vi "Basic RESTws.vi"() -> ()   [LabVIEW 2023]
uses:
  controls/MLA Loops.ctl
  controls/WebSocket VIG States.ctl
  Log/Log_Level.ctl
  API Message/API Message.lvclass
  WebSocket/WebSocket.lvclass
  <vilib>/Utility/config.llb/Write Key (Boolean).vi
  Request/Get Request.vi
  <vilib>/Utility/config.llb/Read Key (Double).vi
  <vilib>/Utility/config.llb/Write Key (String).vi
  <vilib>/addons/control/pid/pid.llb/PID (DBL).vi
  <vilib>/httpClient/POSTBuffer.vi
  Request/Request.lvclass
  Response/Response.lvclass
  MLA/MLA.lvclass
  <vilib>/Utility/config.llb/NI_LVConfig.lvlib
  Log/Log.lvclass
  Server/Server.lvclass
  <vilib>/httpClient/LabVIEWHTTPClient.lvlib
  <vilib>/addons/control/pid/NI_PID_pid.lvlib
panel:
  in  "Get Temperature":bool
  out "Current Temperature":dbl
  in  "Get Target":bool
  out "Current Target":dbl
  in  "Target Set":dbl
  in  "Get Ambient":bool
  in  "Get PIDs":bool
  out "Current Ambient":dbl
  out "Current PIDs":cluster{"P":dbl, "I":dbl, "D":dbl}
  in  "Ambient Set":dbl
  in  "PID Set":cluster{"P":dbl, "I":dbl, "D":dbl}={"P"=1.0, "I"=0.01, "D"=0.0}
  out "Target":dbl=23.0
  out "Ambient":dbl=23.0
  out "PID gains":cluster{"P":dbl, "I":dbl, "D":dbl}={"P"=1.0, "I"=0.01, "D"=0.0}
  out "Temperature Chart":dbl(graph)=23.0
  out "Temperature":dbl=23.0 format="%.2f"
  out "P_heater":dbl format="%.2f"
  in  "REST Send":bool
  in  "REST TX":string
  in  "WS Send":bool
  in  "WS TX":string
  out "All Messages":string
  out "Version":string="1.0.0" caption="V"
  out "Happy":bool=TRUE
  in  "ErrorButton":bool=TRUE
  out "Errors":bool
  out "Status":string="Initializing... "
  # "REST.ws Basic Example"
  # "REST Endpoints"
  # "Process Simulation"
  # "Write Enpoints - change Plant Values"
  # "Read Enpoints - retrieve Plant Values"
  # "All Messages"
  # "www.s5solutions.com"
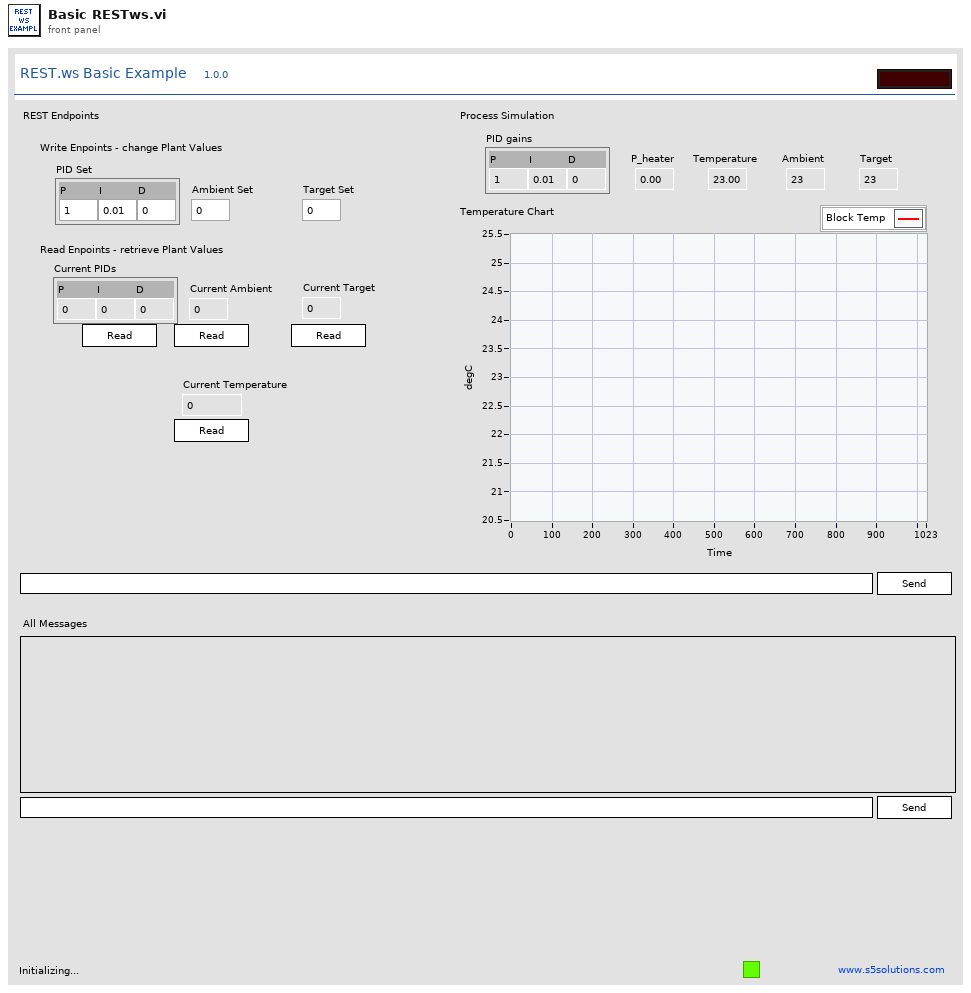
[diagram p1: front panel]
types:
  T1 = cluster{"proportional gain (Kc)":dbl, "integral time (Ti, min)":dbl, "derivative time (Td, min)":dbl}
  T2 = typedef "Log.lvclass/Log_Level.ctl" = enum16{"none", "info", "trace", "warn", "error", "fatal"}
  T3 = typedef "MLA Loops.ctl" = enum16{"Process", "REST", "WS"}
  T4 = typedef "WebSocket VIG States.ctl" = enum16{"Open", "Close", "Send", "Receive", "Check"}
  T5 = enum32{"invalid app kind", "Development System", "Run Time System", "Student Edition", "Embedded LabVIEW", "Evaluation", "Custom"}
  T6 = typedef "NI_LVConfig.lvlib/Config Data RefNum.ctl" = refnum<k1>
  T7 = typedef "LabVIEWHTTPClient.lvlib/ClientHandle.ctl" = refnum<k1>
  T8 = typedef "Request.ctl" = cluster{"Method":string, "URI":string, "Protocol":string, "Raw Path":string, "Query":string, "Fragment":string, "Raw Body":string, "Headers":variant, "Parameters":variant, "Body":variant, "Raw Header":string, "Path":string[]}
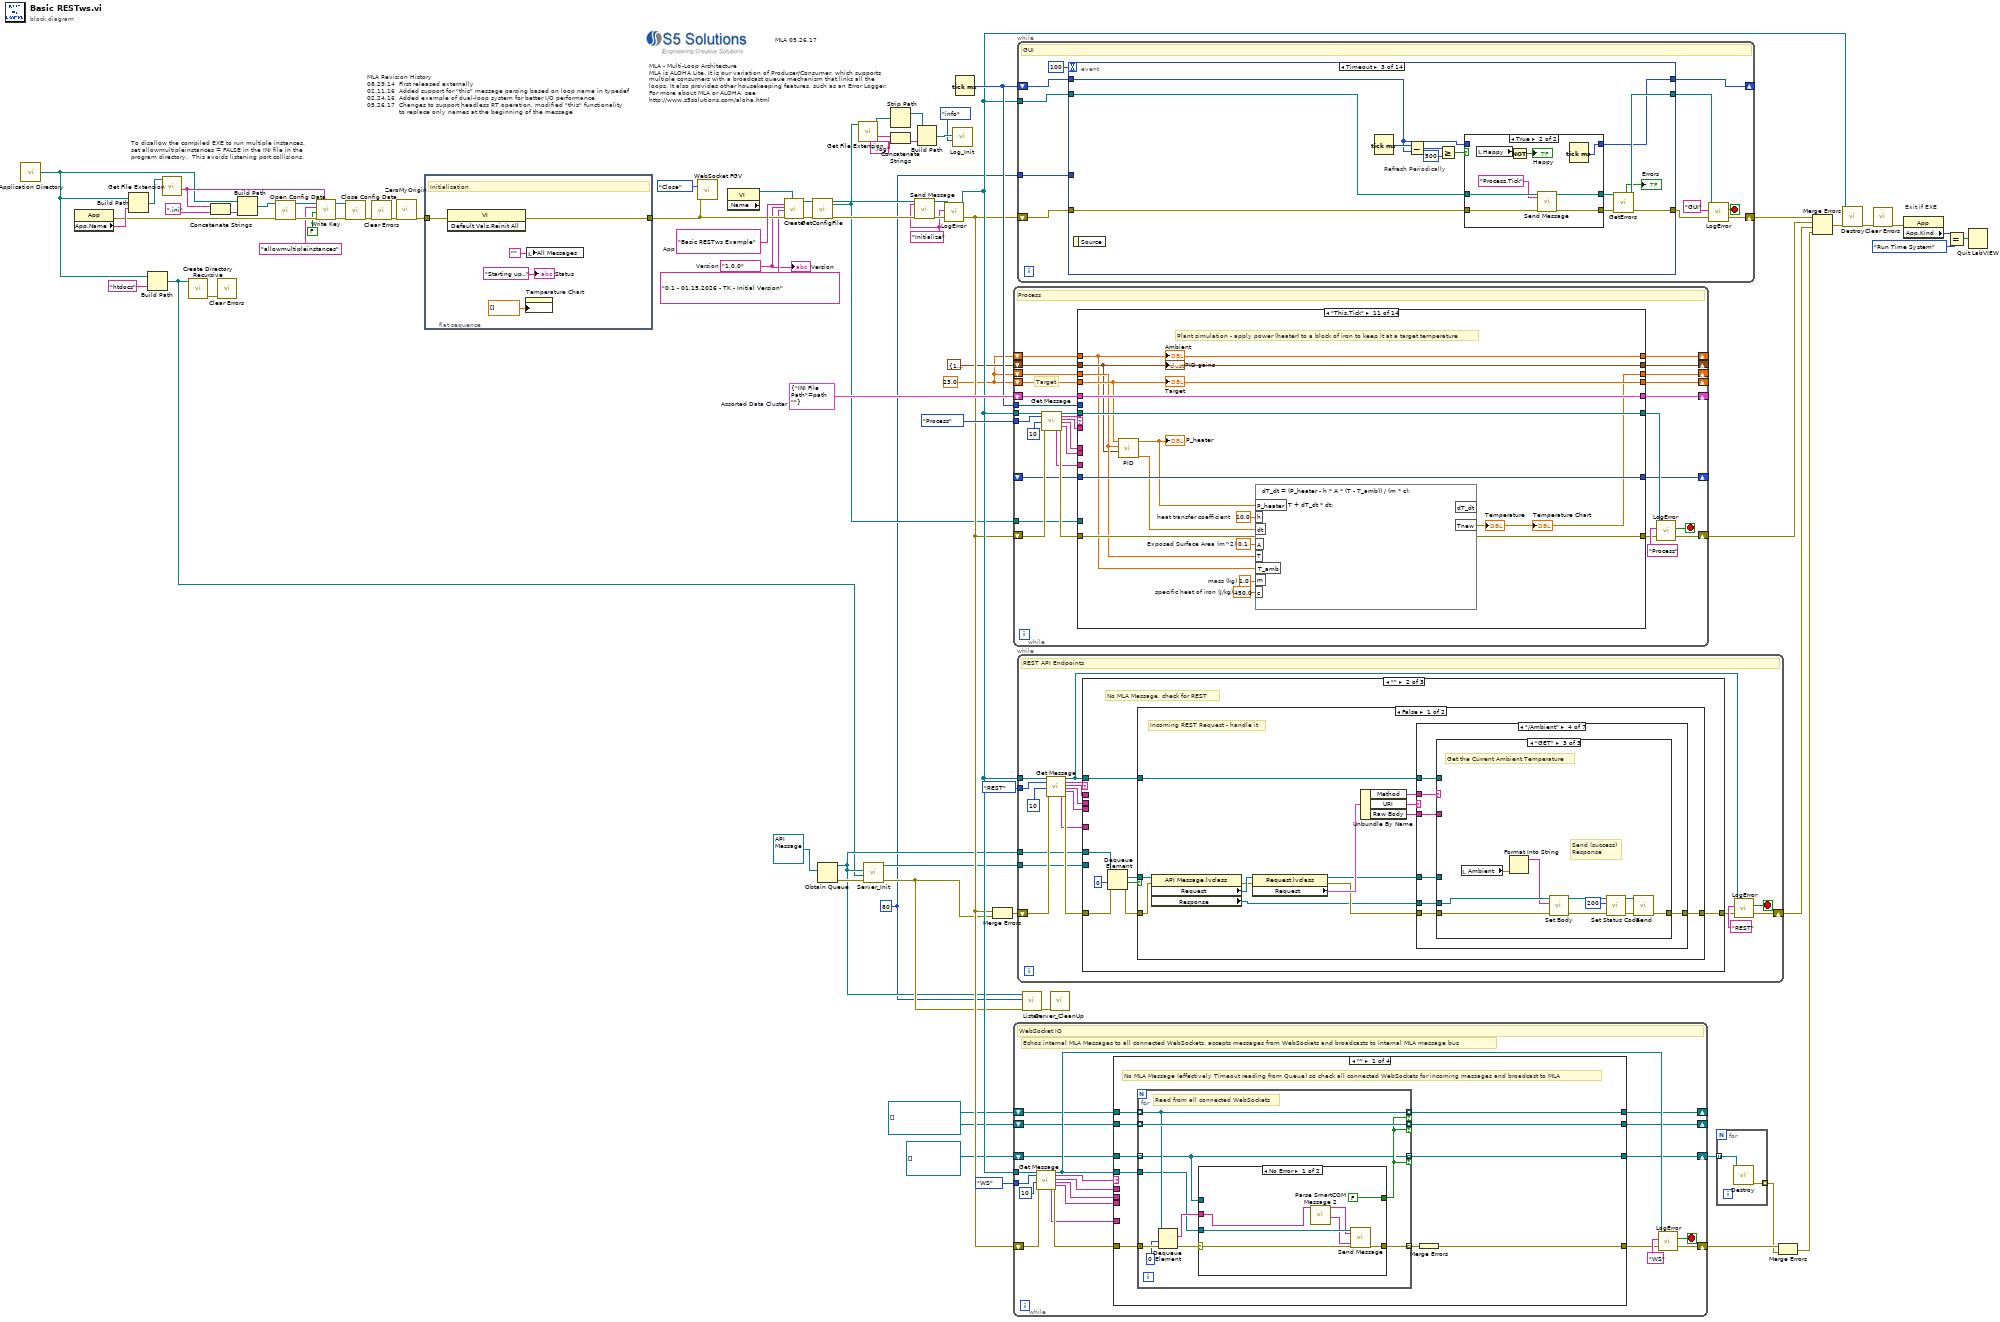
[diagram p0: block diagram]
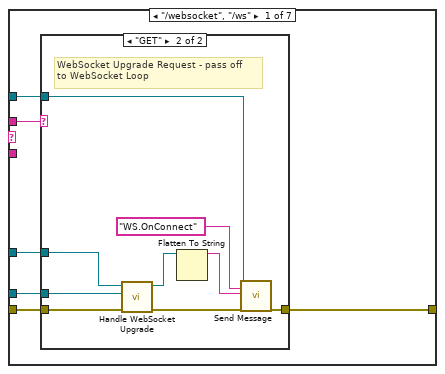
[diagram p3: hidden frame]
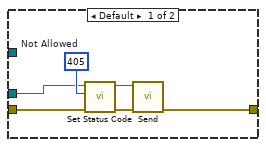
[diagram p4: hidden frame]
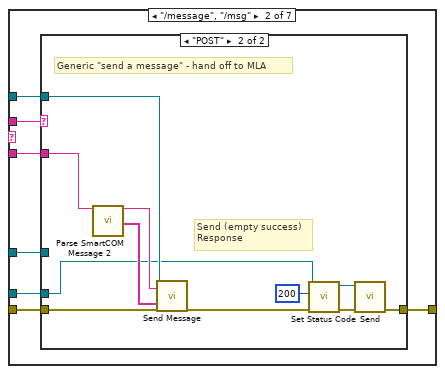
[diagram p5: hidden frame]
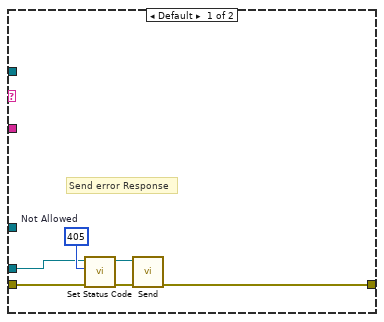
[diagram p6: hidden frame]
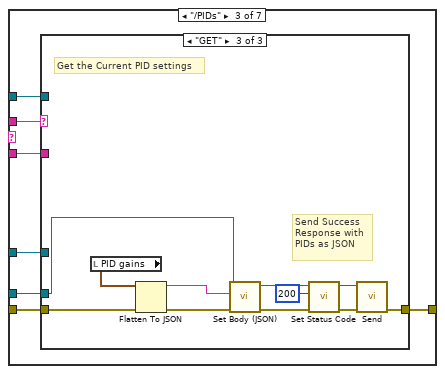
[diagram p7: hidden frame]
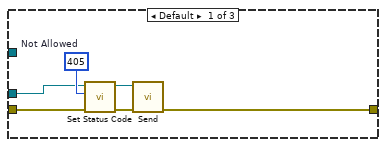
[diagram p8: hidden frame]
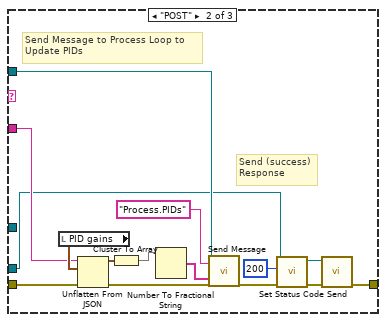
[diagram p9: hidden frame]
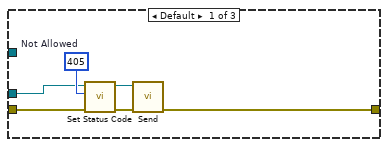
[diagram p10: hidden frame]
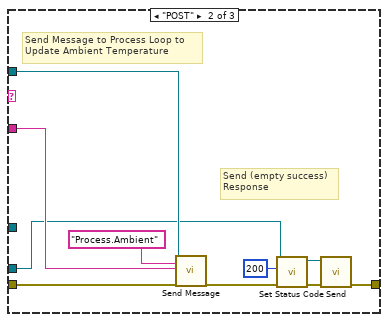
[diagram p11: hidden frame]
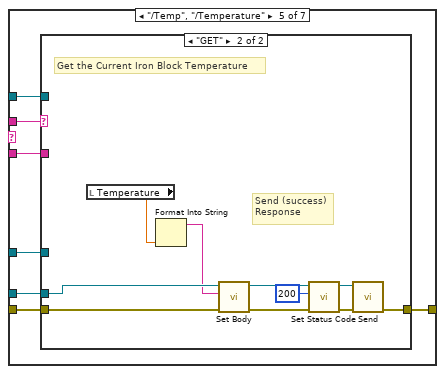
[diagram p12: hidden frame]
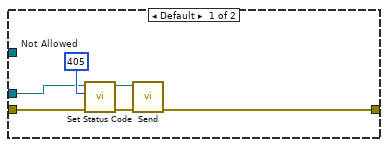
[diagram p13: hidden frame]
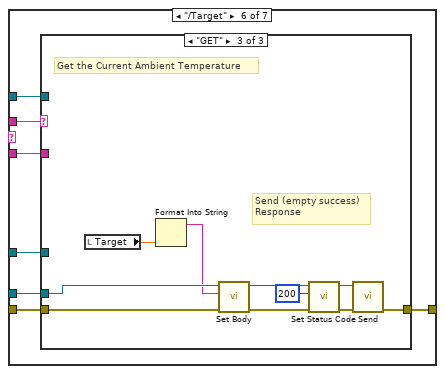
[diagram p14: hidden frame]
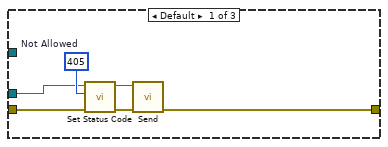
[diagram p15: hidden frame]
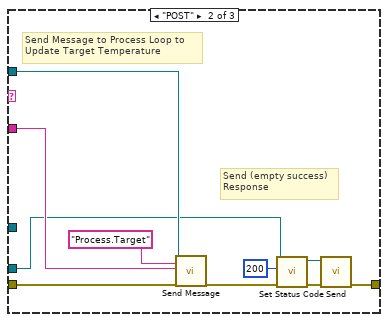
[diagram p16: hidden frame]
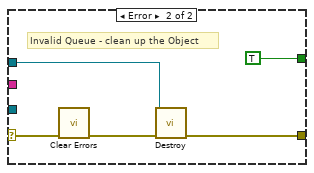
[diagram p20: hidden frame]
diagram:
  w7 = u16 80 ("Listen Port (80)")
  w12 = refnum<queue>[] []
  w5 = 23.0 ("Param 1")
  w42 = "1.0.0"  # Version
  w61 = cluster{"INI File Path":path} {"INI File Path"=path ""}  # Assorted Data Cluster
  w68 = "Basic RESTws Example"  # App
  w9 = "Initialize" ("element")
  # "To disallow the compiled EXE to run multiple instances,\nset allowmultipleinstances = FALSE in the INI file in the\nprogram directory.  This avoids listening port collisions."
  # "MLA Revision History\n08.29.14  First released externally\n02.11.16  Added support for \"this\" message parsing based on loop name in typedef\n02.24.16  Added example of dual-loop system for better I/O performance\n05.26.17  Changes to support headless RT operation, modified \"this\" functionality \n                to replace only names at the beginning of the message"
  # "MLA 05.26.17"
  # "MLA - Multi-Loop Architecture\nMLA is ALOHA Lite. It is our variation of Producer/Consumer, which supports multiple consumers with a broadcast queue mechanism that links all the loops. It also provides other housekeeping features, such as an Error Logger.\nFor more about MLA or ALOHA, see \nhttp://www.s5solutions.com/aloha.html"
  # "Exit if EXE"
  n1 = call <vilib>:"Application Directory.vi"() -> ("Application Directory"=w25:path)
  n2 = property class="App"() -> (error out=w48:errorcluster, "App.Name"=w50:string)  [unwired: 2 in, 1 out]
  n3 = Build Path(base path=w25, name or relative path=w50) -> (appended path=w49:path)
  n4 = Build Path(base path=w25, name or relative path="htdocs" ("section")) -> (appended path=w4:path)
  n5 = call <vilib>:"Get File Extension.vi"("file"=w49) -> ("filename without extension"=w36:string)  [unwired: 6 in, 4 out]
  n6 = call <vilib>:"Create Directory Recursive.vi"("directory"=w4) -> ("error out"=w3:errorcluster)  [unwired: 4 in, 2 out]
  n7 = Concatenate Strings(w36, ".ini" ("section")) -> (w47:string)
  n8 = call <vilib>:"Clear Errors.vi"("error in (no error)"=w3) -> ()  [unwired: 5 in, 2 out]
  n9 = Build Path(base path=w25, name or relative path=w47) -> (appended path=w46:path)
  n10 = call <vilib>:"Open Config Data.vi"("error in (no error)"=w48, "configuration file path"=w46) -> ("error out"=w55:errorcluster, "refnum"=w56:T6)  [unwired: 7 in, 1 out]
  n11 = call-poly <vilib>:"Write Key.vi"("section"=w36, "error in (no error)"=w55, "value"=FALSE, "key"="allowmultipleinstances", "refnum"=w56) -> ("error out"=w58:errorcluster, "refnum out"=w57:T6)  [unwired: 4 in, 1 out]
  n12 = call <vilib>:"Close Config Data.vi"("error in (no error)"=w58, "refnum"=w57) -> ("error out"=w52:errorcluster)  [unwired: 8 in, 1 out]
  n13 = call <vilib>:"Clear Errors.vi"("error in (no error)"=w52) -> ("error out"=w32:errorcluster)  [unwired: 5 in, 1 out]
  n14 = call "ZeroMyOrigin.vi"("error in (no error)"=w32) -> ("error out"=w69:errorcluster)  [unwired: 18 in]
  n15 = flat-sequence "Initialization" {
    tunnel: w69 -> [w74]
    tunnel: [w75] -> w45
    frame #0 {
      # "Initialization"
      n16 = invoke class="VI" method="Default Vals.Reinit All"(error in=w74) -> (error out=w75:errorcluster)  [unwired: 2 in, 2 out]
      n17 = property on="Temperature Chart" class="WFChart (strict)"("History Data"=dbl[] []) -> ()  [unwired: 2 in, 2 out]
      n18 = local write "All Messages"("") -> ()
      "Status" <- "Starting up.." ("Status")
    }
  }
  n19 = call "WebSocket FGV.vi"("Action"=WebSocket_VIG_States."Close", "error in (no error)"=w45) -> ()  [unwired: 8 in, 6 out]
  n20 = property class="VI" props=["Name"]() -> (reference out=w65:refnum<vi>)  [unwired: 2 in, 2 out]
  n21 = call "Create.vi"("Application Name"=w68, "Application Version"=w42, "Revision History"="0.1 - 01.15.2026 - TK - Initial Version" ("Version"), "error in (no error)"=w45, "VI Reference"=w65) -> ("MLA"=w62:refnum<class "MLA.lvclass">, "error out"=w64:errorcluster)  [unwired: 13 in]
  n22 = call-dynamic "GetConfigFile.vi"("MLA"=w62, "error in (no error)"=w64) -> ("MLA"=w63:refnum<class "MLA.lvclass">, "Config File"=w8:path, "error out"=w59:errorcluster)  [unwired: 15 in]
  n23 = Obtain Queue(element data type=refnum<class "API Message.lvclass"> refnum ("API Message.lvclass")) -> (queue out=w20:refnum<queue>, error out=w27:errorcluster)  [unwired: 4 in, 1 out]
  n24 = call <vilib>:"Get File Extension.vi"("file"=w8) -> ("filename without extension"=w31:string, "dup file"=w30:path)  [unwired: 6 in, 3 out]
  n25 = call "Server_Init.vi"("error in (no error)"=w27, "Static Data Folder"=w4, "API Queue"=w20) -> ("error out"=w21:errorcluster, "reference out"=w19:refnum<class "Server.lvclass">)  [unwired: 7 in]
  n26 = Strip Path(path=w30) -> (stripped path=w29:path)  [unwired: 1 out]
  n27 = Concatenate Strings(w31, ".log" ("section")) -> (w35:string)
  n28 = call-dynamic "Send Message.vi"("MLA"=w63, "Message"=w9, "error in (no error)"=w59) -> ("MLA"=w10:refnum<class "MLA.lvclass">, "error out"=w11:errorcluster)  [unwired: 15 in]
  n29 = Build Path(base path=w29, name or relative path=w35) -> (appended path=w34:path)
  n30 = call "LogError.vi"("Error To Log"=w11, "Context (\"Error\")"=w9, "reference in"=w10) -> ("Cleaned Error"=w23:errorcluster, "reference out"=w40:refnum<class "MLA.lvclass">)  [unwired: 2 in, 1 out]
  n31 = call "Log_Init.vi"("Level"=Log_Level."info", "Log File"=w34) -> ()  [unwired: 8 in, 2 out]
  n32 = Tick Count (ms)() -> (millisecond timer value=w60:u32)
  n33 = Merge Errors(w23, w21) -> (w22:errorcluster)
  n34 = while "Process" {
    shift-right: [w103] -> w2
    shift-left: w23 -> [w100]
    tunnel: w40 -> [w101]
    tunnel: MLA_Loops."Process" ("Customize This Typedef =>") -> [w98]
    tunnel: w8 -> [w94]
    shift-right: [w92] -> _
    shift-left: w61 -> [w93]
    tunnel: w60 -> [w91]
    shift-right: [w89] -> _
    shift-left: _ -> [w90]
    shift-right: [w87] -> _
    shift-left: w5 -> [w86]
    shift-right: [w81] -> _
    shift-left: T1 {"proportional gain (Kc)"=1.0, "integral time (Ti, min)"=0.01, "derivative time (Td, min)"=0.0} ("PID gains") -> [w84]
    shift-right: [w82] -> _
    shift-left: w5 -> [w83]
    shift-right: [w80] -> _
    shift-left: w5 -> [w79]
    stop <- w96 stop-if-true
    # "Target"
    # "Process"
    n35 = call-dynamic "Get Message.vi"("MLA"=w101, "Loop"=w98, "Timeout (100mS)"=10, "error in (no error)"=w100) -> ("Raw Message"=w85:string, "MLA"=w97:refnum<class "MLA.lvclass">, "Message"=w104:string, "Param 1"=w108:string, "Param 2"=w107:string, "Params"=w106:string[], "error out"=w99:errorcluster)  [unwired: 8 in, 1 out]
    n36 = case shown="\"This.Tick\"" w104 {
      tunnel: [w116 w124 w134 w146 w155 w156 w170 w188 w208 w216 w231 w240 w249 w261] -> w102
      tunnel: w99 -> [w116 w124 w134 w141 w155 w156 w181 w196 w208 w216 w231 w240 w249 w261]
      tunnel: w108 -> [_ _ _ _ _ _ _ w190 _ _ _ w233 w243 _]
      tunnel: w107 -> [_ _ _ _ _ _ _ _ _ _ _ _ _ _]
      tunnel: w106 -> [_ _ _ _ _ _ _ _ _ _ _ _ _ w254]
      tunnel: w97 -> [w115 w123 w133 w145 w154 w157 w169 w194 w207 w215 w230 w239 w248 w260]
      tunnel: [w115 w123 w133 w144 w154 w157 w169 w187 w207 w215 w230 w239 w248 w260] -> w95
      tunnel: w94 -> [_ _ _ _ _ _ w173 _ _ _ _ _ _ _]
      tunnel: w93 -> [w114 w122 w136 w147 w153 w163 w174 w198 w206 w214 w229 w238 w247 w259]
      tunnel: [w114 w122 w136 w147 w153 w163 w165 w198 w206 w214 w229 w238 w247 w259] -> w92
      tunnel: w91 -> [_ _ _ _ _ _ _ _ _ _ _ _ _ _]
      tunnel: w90 -> [w113 w121 w129 w143 w152 _ w172 w193 w205 w213 w228 w237 w246 w258]
      tunnel: [w113 w121 w129 w143 w152 0 w172 w193 w205 w213 w228 w237 w246 w258] -> w89
      tunnel: [w112 w120 w135 w142 w151 w161 w171 w189 w204 w212 w227 w236 w241 w257] -> w87
      tunnel: w86 -> [w112 w120 w135 w142 w151 w161 w171 w189 w204 w212 w227 w236 _ w257]
      tunnel: w85 -> [_ _ w130 _ _ _ _ _ _ _ _ _ _ _]
      tunnel: w84 -> [w111 w118 w128 w139 w150 w160 w168 w184 w203 w211 w223 w234 w244 w253]
      tunnel: w83 -> [w110 w119 w127 w138 w149 w159 w167 w183 w202 w210 w225 w235 w245 w256]
      tunnel: [w110 w119 w127 w138 w149 w159 w167 w183 w202 w210 w217 w235 w245 w256] -> w82
      tunnel: [w111 w118 w128 w139 w150 w160 w168 w184 w203 w211 w223 w234 w244 w250] -> w81
      tunnel: [w109 w117 w126 w137 w148 w158 w166 w182 w201 w209 w218 w232 w242 w255] -> w80
      tunnel: w79 -> [w109 w117 w126 w137 w148 w158 w166 w182 w201 w209 w218 _ w242 w255]
      frame "-----Miscellaneous-----" {
      }
      frame "" {
        # "No Message - do nothing"
      }
      frame Default {
        # "Unknown/Unhandled message, save it to the message log"
        n37 = local read "All Messages"() -> (w132:string)
        n38 = Concatenate Strings(w132, w130, "\r\n") -> (→"All Messages":string)
      }
      frame "Shutdown" {
        n39 = call "Shutdown.vi"("error in (no error)"=w141) -> ("error out"=w140:errorcluster)  [unwired: 10 in]
        n40 = call-dynamic "Stop.vi"("reference in"=w145, "error in (no error)"=w140) -> ("reference out"=w144:refnum<class "MLA.lvclass">, "error out"=w146:errorcluster)  [unwired: 16 in]
      }
      frame "-----Setup-----" {
      }
      frame "Initialize" {
        n41 = local write "Status"("Initializing... " ("Status")) -> ()
      }
      frame "This.LoadCurrentINI" {
        n42 = call <vilib>:"Open Config Data.vi"("error in (no error)"=w181, "configuration file path"=w173) -> ("error out"=w180:errorcluster, "refnum"=w178:T6)  [unwired: 7 in, 1 out]
        n43 = call-poly <vilib>:"Read Key.vi"("section"="Sim", "error in (no error)"=w180, "key"="Target", "refnum"=w178) -> ("error out"=w177:errorcluster, "refnum out"=w175:T6)  [unwired: 4 in, 2 out]
        n44 = call <vilib>:"Close Config Data.vi"("error in (no error)"=w177, "refnum"=w175) -> ("error out"=w170:errorcluster)  [unwired: 8 in, 1 out]
        n45 = Bundle By Name(cluster=w174, "INI File Path"=w173) -> (w165:cluster{"INI File Path":path})
      }
      frame "This.UpdateINI" {
        n46 = call "Clear Component Lists.vi"("error in (no error)"=w196, "MLA in"=w194) -> ("error out"=w195:errorcluster, "MLA out"=w187:refnum<class "MLA.lvclass">)  [unwired: 8 in]
        n47 = Unbundle By Name(w198) -> ("INI File Path"=w197:path)
        n48 = call <vilib>:"Open Config Data.vi"("error in (no error)"=w195, "configuration file path"=w197) -> ("error out"=w191:errorcluster, "refnum"=w192:T6)  [unwired: 7 in, 1 out]
        n49 = call-poly <vilib>:"Write Key.vi"("section"="Sim", "error in (no error)"=w191, "value"=w190, "key"="Target", "refnum"=w192) -> ("error out"=w185:errorcluster, "refnum out"=w186:T6)  [unwired: 4 in, 1 out]
        n50 = call <vilib>:"Close Config Data.vi"("error in (no error)"=w185, "refnum"=w186) -> ("error out"=w188:errorcluster)  [unwired: 8 in, 1 out]
      }
      frame "-----Menu Functions-----" {
      }
      frame "-----Manage Data-----" {
      }
      frame "This.Tick" {
        w219 = 450.0  # specific heat of iron (J/kg)
        w220 = 1.0  # mass (kg)
        w221 = 0.1  # Exposed Surface Area (m^2)
        w222 = 10.0  # heat transfer coefficient
        # "Plant simulation - apply power (heater) to a block of iron to keep it at a target temperature"
        n51 = call-poly <vilib>:"PID.vi"("PID gains"=w223, "process variable"=w225, "setpoint"=w227) -> ("dt out (s)"=w224:dbl, "output"=w226:dbl)  [unwired: 7 in]
        "P_heater" <- w226
        n52 = formula code="dT_dt = (P_heater - h * A * (T - T_amb)) / (m * c);\n\nTnew = T + dT_dt * dt;"("P_heater"=w226, "h"=w222, "A"=w221, "T"=w225, "T_amb"=w218, "m"=w220, "c"=w219, "dt"=w224) -> ("Tnew"=w217:dbl)  [unwired: 1 out]
        "Temperature Chart" <- w217
        "Temperature" <- w217
        "PID gains" <- w223
        "Ambient" <- w218
        "Target" <- w227
      }
      frame "This.Ambient" {
        n53 = Scan From String(input string=w233) -> (output 1=w232:dbl)  [unwired: 4 in, 3 out]
      }
      frame "This.Target" {
        n54 = Scan From String(input string=w243) -> (output 1=w241:dbl)  [unwired: 4 in, 3 out]
      }
      frame "This.PIDs" {
        n55 = Cluster To Array(cluster=w253) -> (array=w252:dbl[])
        n56 = for {
          tunnel: w254 -> [w264] mode=indexing
          tunnel: w252 -> [w263] mode=indexing
          tunnel: [w262] -> w251 mode=indexing
          n57 = Fract/Exp String To Number(string=w264, default (0 dbl)=w263) -> (number=w262:dbl)  [unwired: 2 in, 1 out]
        }
        n58 = Array To Cluster(array=w251) -> (cluster=w250:cluster{"[0]":dbl, "[1]":dbl, "[2]":dbl})
      }
    }
    n59 = call "LogError.vi"("Error To Log"=w102, "Context (\"Error\")"="Process" ("Context"), "reference in"=w95) -> ("Cleaned Error"=w103:errorcluster, "Stop?"=w96:bool)  [unwired: 2 in, 1 out]
  }
  n60 = while "Send to RT" {
    shift-right: [w284] -> w16
    shift-left: w23 -> [w277]
    tunnel: MLA_Loops."WS" ("Loop") -> [w283]
    tunnel: w40 -> [w282]
    shift-right: [w271] -> w17
    shift-left: refnum<class "WebSocket.lvclass">[] [] -> [w272]
    shift-right: [w266] -> _
    shift-left: w12 -> [w268]
    shift-right: [w267] -> _
    shift-left: w12 -> [w269]
    stop <- w275 stop-if-true
    # "Echos internal MLA Messages to all connected WebSockets, accepts messages from WebSockets and broadcasts to internal MLA message bus"
    # "WebSocket IO"
    n61 = call-dynamic "Get Message.vi"("MLA"=w282, "Loop"=w283, "Timeout (100mS)"=10, "error in (no error)"=w277) -> ("Raw Message"=w274:string, "MLA"=w273:refnum<class "MLA.lvclass">, "Message"=w281:string, "Param 1"=w280:string, "Param 2"=w279:string, "Params"=w278:string[], "error out"=w276:errorcluster)  [unwired: 8 in, 1 out]
    n62 = case shown="\"\"" w281 {
      tunnel: w276 -> [w294 w322 w340 w346]
      tunnel: [w286 w318 w329 w343] -> w265
      tunnel: w280 -> [_ _ w342 w344]
      tunnel: w279 -> [_ _ _ _]
      tunnel: w278 -> [_ _ _ _]
      tunnel: w273 -> [w287 _ _ _]
      tunnel: w274 -> [_ w319 _ _]
      tunnel: w272 -> [w295 w324 w339 w349]
      tunnel: [w293 w324 w338 w350] -> w271
      tunnel: w269 -> [w291 w323 w335 w352]
      tunnel: w268 -> [w290 w321 w334 w351]
      tunnel: [w289 w323 w331 w347] -> w267
      tunnel: [w288 w321 w330 w348] -> w266
      frame "" {
        # "No MLA Message (effectively Timeout reading from Queue) so check all connected WebSockets for incoming messages and broadcast to MLA"
        n63 = for {
          tunnel: w295 -> [w298] mode=indexing
          tunnel: w294 -> [w304]
          tunnel: [w298] -> w293 mode=indexing if=w299
          tunnel: [w300] -> w292 mode=indexing
          tunnel: w291 -> [w303] mode=indexing
          tunnel: w290 -> [w305] mode=indexing
          tunnel: [w303] -> w289 mode=indexing if=w299
          tunnel: [w305] -> w288 mode=indexing if=w299
          tunnel: w287 -> [w296]
          # "Read from all connected WebSockets"
          n64 = Dequeue Element(queue=w303, timeout in ms (-1)=0, error in (no error)=w304) -> (element=w302:string, error out=w301:errorcluster)  [unwired: 2 out]
          n65 = case shown="No Error" w301 {
            selector: w301 -> [w311 w317]
            tunnel: w302 -> [w308 _]
            tunnel: [w310 w314] -> w300
            tunnel: [FALSE TRUE] -> w299
            tunnel: w298 -> [_ w313]
            tunnel: w296 -> [w309 _]
            frame No Error {
              n66 = call "Parse SmartCOM Message 2.vi"("Message"=w308) -> ("Root Message"=w307:string, "All Params"=w306:string[])  [unwired: 10 in, 7 out]
              n67 = call-dynamic "Send Message.vi"("MLA"=w309, "Message"=w307, "Params"=w306, "error in (no error)"=w311) -> ("error out"=w310:errorcluster)  [unwired: 14 in, 1 out]
            }
            frame Error {
              # "Invalid Queue - clean up the Object"
              n68 = call <vilib>:"Clear Errors.vi"("error in (no error)"=w317) -> ("error out"=w315:errorcluster)  [unwired: 5 in, 1 out]
              n69 = call-dynamic "Destroy.vi"("error in (no error)"=w315, "reference in"=w313) -> ("error out"=w314:errorcluster)  [unwired: 8 in, 1 out]
            }
          }
        }
        n70 = Merge Errors(w292) -> (w286:errorcluster)
      }
      frame Default {
        # "Unknown message - send to all connected WebSockets"
        n71 = for {
          tunnel: w322 -> [w327]
          tunnel: w321 -> [w326] mode=indexing
          tunnel: [w328] -> w320 mode=indexing
          tunnel: w319 -> [w325]
          n72 = Enqueue Element(queue=w326, element=w325, error in (no error)=w327) -> (error out=w328:errorcluster)  [unwired: 1 in, 2 out]
        }
        n73 = Merge Errors(w320) -> (w318:errorcluster)
      }
      frame "This.OnConnect" {
        # "Special Message indicating new connection from REST loop"
        n74 = Unflatten From String(type=refnum<class "WebSocket.lvclass"> refnum ("WebSocket"), binary string=w342, error in (no error)=w340) -> (value=w337:refnum<class "WebSocket.lvclass">, error out=w336:errorcluster)  [unwired: 2 in, 1 out]
        n75 = Build Array (concatenate)(w339, w337) -> (w338:refnum<class "WebSocket.lvclass">[])
        n76 = property class="WebSocket"(reference=w337, error in=w336) -> (error out=w329:errorcluster, "properties:FromSocket"=w333:refnum<queue>, "properties:ToSocket"=w332:refnum<queue>)  [unwired: 1 out]
        n77 = Build Array (concatenate)(w335, w333) -> (w331:refnum<queue>[])
        n78 = Build Array (concatenate)(w334, w332) -> (w330:refnum<queue>[])
      }
      frame "This.Transmit" {
        # "Special explicit message (not really needed because of the Default case) to send data to all connected WebSockets"
        n79 = for {
          tunnel: w352 -> [w358] mode=indexing
          tunnel: w351 -> [w354] mode=indexing
          tunnel: [w359] -> w350 mode=indexing
          tunnel: w349 -> [w359] mode=indexing
          tunnel: [w355] -> w348 mode=indexing
          tunnel: [w358] -> w347 mode=indexing
          tunnel: w346 -> [w356]
          tunnel: [w357] -> w345 mode=indexing
          tunnel: w344 -> [w353]
          n80 = Enqueue Element(queue=w354, element=w353, error in (no error)=w356) -> (queue out=w355:refnum<queue>, error out=w357:errorcluster)  [unwired: 1 in, 1 out]
        }
        n81 = Merge Errors(w345) -> (w343:errorcluster)
      }
    }
    n82 = call "LogError.vi"("Error To Log"=w265, "Context (\"Error\")"="WS" ("Context"), "reference in"=w273) -> ("Cleaned Error"=w284:errorcluster, "Stop?"=w275:bool)  [unwired: 2 in, 1 out]
  }
  n83 = while "GUI" {
    shift-right: [w368] -> w73
    shift-left: w23 -> [w370]
    shift-right: [w361] -> _
    shift-left: w60 -> [w366]
    tunnel: w40 -> [w363]
    tunnel: w7 -> [w360]
    stop <- w365 stop-if-true
    # "GUI"
    n84 = event shown="[2] Timeout" {
      selector: _ -> [_ _ _ _ _ _ _ _ _ _ _ _ _ _]
      dyn-events: _ -> [_ _ _ _ _ _ _ _ _ _ _ _ _ _]
      timeout: 100 -> [_ _ _ _ _ _ _ _ _ _ _ _ _ _]
      tunnel: w370 -> [w371 w382 w394 w426 w435 w441 w461 w476 w491 w506 w520 w534 w548 w559]
      tunnel: [w373 w380 w403 w426 w434 w442 w455 w471 w486 w501 w521 w535 w549 w558] -> w367
      tunnel: w366 -> [w376 w383 w395 w425 w436 w451 w467 w482 w497 w512 w527 w541 w555 w557]
      tunnel: [w376 w383 w397 w425 w436 w451 w467 w482 w497 w512 w527 w541 w555 w557] -> w361
      tunnel: w363 -> [w372 w381 w391 w424 w433 w448 w466 w481 w496 w511 w526 w540 w554 w556]
      tunnel: [w374 w379 w398 w424 w432 w448 w466 w481 w496 w511 w526 w540 w554 w556] -> w362
      tunnel: w360 -> [_ _ _ _ _ w439 w459 w474 w489 w504 w519 w533 w547 _]
      event Panel Close? {
        n85 = event-data() -> ()  [unwired: 1 in, 1 out]
        n86 = call-dynamic "Send Message.vi"("MLA"=w372, "Message"="Shutdown" ("element"), "error in (no error)"=w371) -> ("MLA"=w374:refnum<class "MLA.lvclass">, "error out"=w373:errorcluster)  [unwired: 15 in]
        n87 = event-data("Discard?"=TRUE) -> ()  [unwired: 1 in, 1 out]
      }
      event Menu Selection (User) {
        n88 = event-data() -> ("ItemTag"=w378:string)  [unwired: 1 in]
        n89 = disable-structure shown="Enabled" {
          disable-tunnel: w382 -> [w388 w389]
          disable-tunnel: w381 -> [w387 w390]
          disable-tunnel: [w386 w389] -> w380
          disable-tunnel: [w385 w390] -> w379
          disable-tunnel: w378 -> [w384 _]
          frame Enabled {
            n90 = call "Read Menu Action.vi"("error in (no error)"=w388, "ItemTag"=w384, "MLA in"=w387) -> ("error out"=w386:errorcluster, "MLA out"=w385:refnum<class "MLA.lvclass">)  [unwired: 7 in]
          }
          frame Disabled {
          }
        }
      }
      event Timeout {
        # "Refresh Periodically"
        n91 = event-data() -> ()  [unwired: 1 in, 1 out]
        n92 = Tick Count (ms)() -> (millisecond timer value=w400:u32)
        n93 = Subtract(x=w400, y=w395) -> (x-y=w401:u32)
        n94 = Greater Or Equal?(x=w401, y=u32 500) -> (x >= y?=w399:bool)
        n95 = case shown="True" w399 {
          tunnel: w395 -> [w406 _]
          tunnel: [w406 w412] -> w397
          tunnel: w394 -> [w404 w411]
          tunnel: [w404 w410] -> w393
          tunnel: w391 -> [w405 w409]
          tunnel: [w405 w408] -> w392
          frame False {
          }
          frame True {
            n96 = local read "Happy"() -> (w413:bool)
            n97 = Not(x=w413) -> (.not. x?=→"Happy":bool)
            n98 = call-dynamic "Send Message.vi"("MLA"=w409, "Message"="Process.Tick", "error in (no error)"=w411) -> ("MLA"=w408:refnum<class "MLA.lvclass">, "error out"=w410:errorcluster)  [unwired: 15 in]
            n99 = Tick Count (ms)() -> (millisecond timer value=w412:u32)
          }
        }
        n100 = call-dynamic "GetErrors.vi"("error in (no error)"=w393, "reference in"=w392) -> ("error out"=w403:errorcluster, "reference out"=w398:refnum<class "MLA.lvclass">, "Uncleared Errors"=→"Errors":bool)  [unwired: 4 in, 3 out]
      }
      event Key Down {
        n101 = event-data() -> ("Char"=w421:i16, "PlatMods.Ctrl"=w422:bool, "PlatMods.Shift"=w423:bool)  [unwired: 1 in]
        n102 = String To Byte Array(string="B") -> (unsigned byte array=w419:u8[])
        n103 = Index Array(array=w419) -> (element=w418:u8)  [unwired: 1 in]
        n104 = And(x=w422, y=w423) -> (x .and. y?=w416:bool)
        n105 = Equal?(x=w418, y=w421) -> (x = y?=w417:bool)
        n106 = And(x=w417, y=w416) -> (x .and. y?=w415:bool)
        n107 = case shown="True" w415 {
          frame False {
          }
          frame True {
            n108 = property class="VI"("BDWin.Open"=TRUE ("Block Diagram Window:Open")) -> ()  [unwired: 2 in, 2 out]
          }
        }
      }
      event "WS Send": Value Change {
        n109 = event-data() -> ()  [unwired: 1 in, 1 out]
        n110 = String Length(string="WS TX") -> (length=w428:i32)
        n111 = call-dynamic "Send Message.vi"("MLA"=w433, "Message"="WS.Transmit" ("element"), "Param 1"="WS TX", "error in (no error)"=w435) -> ("MLA"=w432:refnum<class "MLA.lvclass">, "error out"=w434:errorcluster)  [unwired: 14 in]
        n112 = property on="WS TX" class="Str"("Text.Selection End"=u32 0 ("Text.Selection:End"), "Text.Selection Start"=w428) -> ()  [unwired: 2 in, 2 out]
      }
      event "REST Send": Value Change {
        n113 = event-data() -> ()  [unwired: 1 in, 1 out]
        n114 = Format Into String(format string="http://localhost:%d/msg", error in=w441, w439) -> (resulting string=w437:string, error out=w440:errorcluster)  [unwired: 1 in]
        n115 = call <vilib>:"OpenHandle.vi"("error in (no error)"=w440) -> ("client handle out"=w446:T7, "error out"=w447:errorcluster)  [unwired: 13 in]
        n116 = call-poly <vilib>:"POST.vi"("client handle"=w446, "url"=w437, "buffer"="REST TX", "error in (no error)"=w447) -> ("client handle out"=w443:T7, "error out"=w444:errorcluster)  [unwired: 8 in, 2 out]
        n117 = call <vilib>:"CloseHandle.vi"("client handle"=w443, "error in (no error)"=w444) -> ("error out"=w442:errorcluster)  [unwired: 13 in]
        n118 = String Length(string="REST TX") -> (length=w449:i32)
        n119 = property on="REST TX" class="Str"("Text.Selection End"=u32 0 ("Text.Selection:End"), "Text.Selection Start"=w449) -> ()  [unwired: 2 in, 2 out]
      }
      event "Get PIDs": Value Change {
        n120 = event-data() -> ()  [unwired: 1 in, 1 out]
        n121 = Format Into String(format string="http://localhost:%d/PIDs", error in=w461, w459) -> (resulting string=w457:string, error out=w460:errorcluster)  [unwired: 1 in]
        n122 = call <vilib>:"OpenHandle.vi"("error in (no error)"=w460) -> ("client handle out"=w464:T7, "error out"=w465:errorcluster)  [unwired: 13 in]
        n123 = call <vilib>:"GET.vi"("client handle"=w464, "url"=w457, "error in (no error)"=w465) -> ("client handle out"=w462:T7, "body"=w452:string, "error out"=w463:errorcluster)  [unwired: 9 in, 1 out]
        n124 = local read "Current PIDs"() -> (w453:cluster{"P":dbl, "I":dbl, "D":dbl})
        n125 = call <vilib>:"CloseHandle.vi"("client handle"=w462, "error in (no error)"=w463) -> ("error out"=w456:errorcluster)  [unwired: 13 in]
        n126 = Unflatten From JSON(JSON string=w452, type and defaults=w453, error in (no error)=w456) -> (value=→"Current PIDs":cluster{"P":dbl, "I":dbl, "D":dbl}, error out=w455:errorcluster)  [unwired: 4 in]
      }
      event "Get Ambient": Value Change {
        n127 = event-data() -> ()  [unwired: 1 in, 1 out]
        n128 = Format Into String(format string="http://localhost:%d/Ambient", error in=w476, w474) -> (resulting string=w472:string, error out=w475:errorcluster)  [unwired: 1 in]
        n129 = call <vilib>:"OpenHandle.vi"("error in (no error)"=w475) -> ("client handle out"=w479:T7, "error out"=w480:errorcluster)  [unwired: 13 in]
        n130 = call <vilib>:"GET.vi"("client handle"=w479, "url"=w472, "error in (no error)"=w480) -> ("client handle out"=w477:T7, "body"=w470:string, "error out"=w478:errorcluster)  [unwired: 9 in, 1 out]
        n131 = call <vilib>:"CloseHandle.vi"("client handle"=w477, "error in (no error)"=w478) -> ("error out"=w471:errorcluster)  [unwired: 13 in]
        n132 = local read "Current Ambient"() -> (w468:dbl)
        n133 = Fract/Exp String To Number(string=w470, default (0 dbl)=w468) -> (number=→"Current Ambient":dbl)  [unwired: 2 in, 1 out]
      }
      event "Get Target": Value Change {
        n134 = event-data() -> ()  [unwired: 1 in, 1 out]
        n135 = Format Into String(format string="http://localhost:%d/Target", error in=w491, w489) -> (resulting string=w487:string, error out=w490:errorcluster)  [unwired: 1 in]
        n136 = call <vilib>:"OpenHandle.vi"("error in (no error)"=w490) -> ("client handle out"=w494:T7, "error out"=w495:errorcluster)  [unwired: 13 in]
        n137 = call <vilib>:"GET.vi"("client handle"=w494, "url"=w487, "error in (no error)"=w495) -> ("client handle out"=w492:T7, "body"=w485:string, "error out"=w493:errorcluster)  [unwired: 9 in, 1 out]
        n138 = call <vilib>:"CloseHandle.vi"("client handle"=w492, "error in (no error)"=w493) -> ("error out"=w486:errorcluster)  [unwired: 13 in]
        n139 = local read "Current Target"() -> (w484:dbl)
        n140 = Fract/Exp String To Number(string=w485, default (0 dbl)=w484) -> (number=→"Current Target":dbl)  [unwired: 2 in, 1 out]
      }
      event "Get Temperature": Value Change {
        n141 = event-data() -> ()  [unwired: 1 in, 1 out]
        n142 = Format Into String(format string="http://localhost:%d/Temp", error in=w506, w504) -> (resulting string=w502:string, error out=w505:errorcluster)  [unwired: 1 in]
        n143 = call <vilib>:"OpenHandle.vi"("error in (no error)"=w505) -> ("client handle out"=w509:T7, "error out"=w510:errorcluster)  [unwired: 13 in]
        n144 = call <vilib>:"GET.vi"("client handle"=w509, "url"=w502, "error in (no error)"=w510) -> ("client handle out"=w507:T7, "body"=w500:string, "error out"=w508:errorcluster)  [unwired: 9 in, 1 out]
        n145 = local read "Current Temperature"() -> (w499:dbl)
        n146 = call <vilib>:"CloseHandle.vi"("client handle"=w507, "error in (no error)"=w508) -> ("error out"=w501:errorcluster)  [unwired: 13 in]
        n147 = Fract/Exp String To Number(string=w500, default (0 dbl)=w499) -> (number=→"Current Temperature":dbl)  [unwired: 2 in, 1 out]
      }
      event "PID Set": Value Change {
        n148 = event-data() -> ()  [unwired: 1 in, 3 out]
        n149 = Format Into String(format string="http://localhost:%d/PIDs", error in=w520, w519) -> (resulting string=w517:string, error out=w516:errorcluster)  [unwired: 1 in]
        n150 = Flatten To JSON(anything="PID Set", error in (no error)=w516) -> (JSON string=w514:string, 11:w515:errorcluster)  [unwired: 1 in]
        n151 = call <vilib>:"OpenHandle.vi"("error in (no error)"=w515) -> ("client handle out"=w524:T7, "error out"=w525:errorcluster)  [unwired: 13 in]
        n152 = call-poly <vilib>:"POST.vi"("client handle"=w524, "url"=w517, "buffer"=w514, "error in (no error)"=w525) -> ("client handle out"=w522:T7, "error out"=w523:errorcluster)  [unwired: 8 in, 2 out]
        n153 = call <vilib>:"CloseHandle.vi"("client handle"=w522, "error in (no error)"=w523) -> ("error out"=w521:errorcluster)  [unwired: 13 in]
      }
      event "Ambient Set": Value Change {
        n154 = event-data() -> ()  [unwired: 1 in, 3 out]
        n155 = Format Into String(format string="http://localhost:%d/Ambient", error in=w534, w533) -> (resulting string=w531:string, error out=w530:errorcluster)  [unwired: 1 in]
        n156 = Format Into String("Ambient Set") -> (resulting string=w528:string)  [unwired: 3 in, 1 out]
        n157 = call <vilib>:"OpenHandle.vi"("error in (no error)"=w530) -> ("client handle out"=w538:T7, "error out"=w539:errorcluster)  [unwired: 13 in]
        n158 = call-poly <vilib>:"POST.vi"("client handle"=w538, "url"=w531, "buffer"=w528, "error in (no error)"=w539) -> ("client handle out"=w536:T7, "error out"=w537:errorcluster)  [unwired: 8 in, 2 out]
        n159 = call <vilib>:"CloseHandle.vi"("client handle"=w536, "error in (no error)"=w537) -> ("error out"=w535:errorcluster)  [unwired: 13 in]
      }
      event "Target Set": Value Change {
        n160 = event-data() -> ()  [unwired: 1 in, 3 out]
        n161 = Format Into String(format string="http://localhost:%d/Target", error in=w548, w547) -> (resulting string=w545:string, error out=w544:errorcluster)  [unwired: 1 in]
        n162 = Format Into String("Target Set") -> (resulting string=w543:string)  [unwired: 3 in, 1 out]
        n163 = call <vilib>:"OpenHandle.vi"("error in (no error)"=w544) -> ("client handle out"=w552:T7, "error out"=w553:errorcluster)  [unwired: 13 in]
        n164 = call-poly <vilib>:"POST.vi"("client handle"=w552, "url"=w545, "buffer"=w543, "error in (no error)"=w553) -> ("client handle out"=w550:T7, "error out"=w551:errorcluster)  [unwired: 8 in, 2 out]
        n165 = call <vilib>:"CloseHandle.vi"("client handle"=w550, "error in (no error)"=w551) -> ("error out"=w549:errorcluster)  [unwired: 13 in]
      }
      event "ErrorButton": Value Change {
        n166 = event-data() -> ()  [unwired: 1 in, 1 out]
        n167 = call-dynamic "ShowErrorDialog.vi"("reference in"=w556, "error in (no error)"=w559) -> ("error out"=w558:errorcluster)  [unwired: 16 in, 1 out]
      }
    }
    n168 = call "LogError.vi"("Error To Log"=w367, "Context (\"Error\")"="GUI" ("Context"), "reference in"=w362) -> ("Cleaned Error"=w368:errorcluster, "Stop?"=w365:bool)  [unwired: 2 in, 1 out]
  }
  n169 = while "Send to RT" {
    shift-right: [w575] -> w38
    shift-left: w22 -> [w567]
    tunnel: MLA_Loops."REST" ("Loop") -> [w573]
    tunnel: w40 -> [w572]
    tunnel: w19 -> [w561]
    tunnel: w20 -> [w560]
    stop <- w565 stop-if-true
    # "REST API Endpoints"
    n170 = call-dynamic "Get Message.vi"("MLA"=w572, "Loop"=w573, "Timeout (100mS)"=10, "error in (no error)"=w567) -> ("Raw Message"=w564:string, "MLA"=w563:refnum<class "MLA.lvclass">, "Message"=w571:string, "Param 1"=w570:string, "Param 2"=w569:string, "Params"=w568:string[], "error out"=w566:errorcluster)  [unwired: 8 in, 1 out]
    n171 = case shown="\"\"" w571 {
      tunnel: w566 -> [w577 w585 w774]
      tunnel: [w577 w581 w774] -> w574
      tunnel: w570 -> [_ _ _]
      tunnel: w569 -> [_ _ _]
      tunnel: w568 -> [_ _ _]
      tunnel: w563 -> [_ w579 _]
      tunnel: w564 -> [_ _ _]
      tunnel: w561 -> [_ _ _]
      tunnel: w560 -> [_ w584 _]
      frame Default {
      }
      frame "" {
        # "No MLA Message, check for REST"
        n172 = Dequeue Element(queue=w584, timeout in ms (-1)=0, error in (no error)=w585) -> (element=w580:refnum<class "API Message.lvclass">, timed out?=w583:bool, error out=w582:errorcluster)  [unwired: 1 out]
        n173 = case shown="False" w583 {
          tunnel: w582 -> [w597 w773]
          tunnel: [w591 w773] -> w581
          tunnel: w580 -> [w598 _]
          tunnel: w579 -> [w587 _]
          frame False {
            # "Incoming REST Request - handle it"
            n174 = property class="API Message.lvclass"(reference=w598, error in=w597) -> (error out=w595:errorcluster, "Request"=w596:refnum<class "Request.lvclass">, "Response"=w588:refnum<class "Response.lvclass">)  [unwired: 1 out]
            n175 = property class="Request.lvclass"(reference=w596, error in=w595) -> (reference out=w589:refnum<class "Request.lvclass">, error out=w592:errorcluster, "Request"=w594:T8)
            n176 = Unbundle By Name(w594) -> ("Method"=w590:string, "URI"=w593:string, "Raw Body"=w586:string)
            n177 = case shown="\"/Ambient\"" w593 {
              tunnel: w592 -> [w603 w625 w649 w688 w721 w744 w772]
              tunnel: [w604 w626 w650 w689 w722 w745 w772] -> w591
              tunnel: w590 -> [w600 w622 w646 w685 w718 w741 _]
              tunnel: w589 -> [w602 w624 w648 w687 w720 w743 _]
              tunnel: w588 -> [w601 w623 w647 w686 w719 w742 _]
              tunnel: w587 -> [w599 w621 w645 w684 w717 w740 _]
              tunnel: w586 -> [_ w620 w644 w683 w716 w739 _]
              frame "/websocket", "/ws" {
                n178 = case shown="\"GET\"" w600 {
                  tunnel: [w605 w614] -> w604
                  tunnel: w603 -> [w609 w618]
                  tunnel: w602 -> [_ w617]
                  tunnel: w601 -> [w608 w616]
                  tunnel: w599 -> [_ w613]
                  frame Default {
                    w610 = u16 405  # Not Allowed
                    n179 = call "Set Status Code.vi"("error in (no error)"=w609, "Status Code"=w610, "Response in"=w608) -> ("error out"=w606:errorcluster, "Response out"=w607:refnum<class "Response.lvclass">)  [unwired: 7 in]
                    n180 = call "Send.vi"("error in (no error)"=w606, "Response in"=w607) -> ("error out"=w605:errorcluster)  [unwired: 9 in]
                  }
                  frame "GET" {
                    # "WebSocket Upgrade Request - pass off\nto WebSocket Loop"
                    n181 = call "Handle WebSocket Upgrade.vi"("error in (no error)"=w618, "Response.lvclass"=w616, "Request.lvclass"=w617) -> ("error out"=w619:errorcluster, "WebSocket"=w615:refnum<class "WebSocket.lvclass">)  [unwired: 7 in]
                    n182 = Flatten To String(anything=w615) -> (data string=w612:string)  [unwired: 3 in, 2 out]
                    n183 = call-dynamic "Send Message.vi"("MLA"=w613, "Message"="WS.OnConnect", "Param 1"=w612, "error in (no error)"=w619) -> ("error out"=w614:errorcluster)  [unwired: 14 in, 1 out]
                  }
                }
              }
              frame "/message", "/msg" {
                n184 = case shown="\"POST\"" w622 {
                  tunnel: [w627 w642] -> w626
                  tunnel: w625 -> [w631 w641]
                  tunnel: w624 -> [_ _]
                  tunnel: w623 -> [w630 w633]
                  tunnel: w621 -> [_ w643]
                  tunnel: w620 -> [_ w640]
                  frame Default {
                    w632 = u16 405  # Not Allowed
                    # "Send error Response"
                    n185 = call "Set Status Code.vi"("error in (no error)"=w631, "Status Code"=w632, "Response in"=w630) -> ("error out"=w628:errorcluster, "Response out"=w629:refnum<class "Response.lvclass">)  [unwired: 7 in]
                    n186 = call "Send.vi"("error in (no error)"=w628, "Response in"=w629) -> ("error out"=w627:errorcluster)  [unwired: 9 in]
                  }
                  frame "POST" {
                    # "Send (empty success)\nResponse"
                    # "Generic \"send a message\" - hand off to MLA"
                    n187 = call "Parse SmartCOM Message 2.vi"("Message"=w640) -> ("Root Message"=w639:string, "All Params"=w638:string[])  [unwired: 10 in, 7 out]
                    n188 = call-dynamic "Send Message.vi"("MLA"=w643, "Message"=w639, "Params"=w638, "error in (no error)"=w641) -> ("error out"=w636:errorcluster)  [unwired: 14 in, 1 out]
                    n189 = call "Set Status Code.vi"("error in (no error)"=w636, "Status Code"=u16 200, "Response in"=w633) -> ("error out"=w635:errorcluster, "Response out"=w634:refnum<class "Response.lvclass">)  [unwired: 7 in]
                    n190 = call "Send.vi"("error in (no error)"=w635, "Response in"=w634) -> ("error out"=w642:errorcluster)  [unwired: 9 in]
                  }
                }
              }
              frame "/PIDs" {
                n191 = case shown="\"GET\"" w646 {
                  tunnel: [w651 w664 w681] -> w650
                  tunnel: w649 -> [w655 w662 w680]
                  tunnel: w648 -> [_ _ _]
                  tunnel: w647 -> [w654 w657 w678]
                  tunnel: w645 -> [_ w671 _]
                  tunnel: w644 -> [_ w663 _]
                  frame Default {
                    w656 = u16 405  # Not Allowed
                    n192 = call "Set Status Code.vi"("error in (no error)"=w655, "Status Code"=w656, "Response in"=w654) -> ("error out"=w652:errorcluster, "Response out"=w653:refnum<class "Response.lvclass">)  [unwired: 7 in]
                    n193 = call "Send.vi"("error in (no error)"=w652, "Response in"=w653) -> ("error out"=w651:errorcluster)  [unwired: 9 in]
                  }
                  frame "POST" {
                    # "Send (success)\nResponse"
                    # "Send Message to Process Loop to\nUpdate PIDs"
                    n194 = local read "PID gains"() -> (w669:cluster{"P":dbl, "I":dbl, "D":dbl})
                    n195 = Unflatten From JSON(JSON string=w663, type and defaults=w669, error in (no error)=w662) -> (value=w668:cluster{"P":dbl, "I":dbl, "D":dbl}, error out=w670:errorcluster)  [unwired: 4 in]
                    n196 = Cluster To Array(cluster=w668) -> (array=w667:dbl[])
                    n197 = Number To Fractional String(number=w667) -> (F-format string=w666:string[])  [unwired: 3 in]
                    n198 = call-dynamic "Send Message.vi"("MLA"=w671, "Message"="Process.PIDs", "Params"=w666, "error in (no error)"=w670) -> ("error out"=w660:errorcluster)  [unwired: 14 in, 1 out]
                    n199 = call "Set Status Code.vi"("error in (no error)"=w660, "Status Code"=u16 200, "Response in"=w657) -> ("error out"=w658:errorcluster, "Response out"=w659:refnum<class "Response.lvclass">)  [unwired: 7 in]
                    n200 = call "Send.vi"("error in (no error)"=w658, "Response in"=w659) -> ("error out"=w664:errorcluster)  [unwired: 9 in]
                  }
                  frame "GET" {
                    # "Send Success\nResponse with\nPIDs as JSON"
                    # "Get the Current PID settings"
                    n201 = local read "PID gains"() -> (w682:cluster{"P":dbl, "I":dbl, "D":dbl})
                    n202 = Flatten To JSON(anything=w682, error in (no error)=w680) -> (JSON string=w677:string, 11:w679:errorcluster)  [unwired: 1 in]
                    n203 = call "Set Body (JSON).vi"("error in (no error)"=w679, "Body (as JSON)"=w677, "Response in"=w678) -> ("error out"=w675:errorcluster, "Response out"=w674:refnum<class "Response.lvclass">)  [unwired: 7 in]
                    n204 = call "Set Status Code.vi"("error in (no error)"=w675, "Status Code"=u16 200, "Response in"=w674) -> ("error out"=w672:errorcluster, "Response out"=w673:refnum<class "Response.lvclass">)  [unwired: 7 in]
                    n205 = call "Send.vi"("error in (no error)"=w672, "Response in"=w673) -> ("error out"=w681:errorcluster)  [unwired: 9 in]
                  }
                }
              }
              frame "/Ambient" {
                n206 = case shown="\"GET\"" w685 {
                  tunnel: [w690 w702 w715] -> w689
                  tunnel: w688 -> [w694 w700 w714]
                  tunnel: w687 -> [_ _ _]
                  tunnel: w686 -> [w693 w697 w713]
                  tunnel: w684 -> [_ w705 _]
                  tunnel: w683 -> [_ w701 _]
                  frame Default {
                    w695 = u16 405  # Not Allowed
                    n207 = call "Set Status Code.vi"("error in (no error)"=w694, "Status Code"=w695, "Response in"=w693) -> ("error out"=w691:errorcluster, "Response out"=w692:refnum<class "Response.lvclass">)  [unwired: 7 in]
                    n208 = call "Send.vi"("error in (no error)"=w691, "Response in"=w692) -> ("error out"=w690:errorcluster)  [unwired: 9 in]
                  }
                  frame "POST" {
                    # "Send (empty success)\nResponse"
                    # "Send Message to Process Loop to\nUpdate Ambient Temperature"
                    n209 = call-dynamic "Send Message.vi"("MLA"=w705, "Message"="Process.Ambient", "Param 1"=w701, "error in (no error)"=w700) -> ("error out"=w703:errorcluster)  [unwired: 14 in, 1 out]
                    n210 = call "Set Status Code.vi"("error in (no error)"=w703, "Status Code"=u16 200, "Response in"=w697) -> ("error out"=w699:errorcluster, "Response out"=w698:refnum<class "Response.lvclass">)  [unwired: 7 in]
                    n211 = call "Send.vi"("error in (no error)"=w699, "Response in"=w698) -> ("error out"=w702:errorcluster)  [unwired: 9 in]
                  }
                  frame "GET" {
                    # "Send (success)\nResponse"
                    # "Get the Current Ambient Temperature"
                    n212 = local read "Ambient"() -> (w712:dbl)
                    n213 = Format Into String(w712) -> (resulting string=w711:string)  [unwired: 3 in, 1 out]
                    n214 = call "Set Body.vi"("error in (no error)"=w714, "Body"=w711, "Response in"=w713) -> ("error out"=w707:errorcluster, "Response out"=w708:refnum<class "Response.lvclass">)  [unwired: 7 in]
                    n215 = call "Set Status Code.vi"("error in (no error)"=w707, "Status Code"=u16 200, "Response in"=w708) -> ("error out"=w706:errorcluster, "Response out"=w709:refnum<class "Response.lvclass">)  [unwired: 7 in]
                    n216 = call "Send.vi"("error in (no error)"=w706, "Response in"=w709) -> ("error out"=w715:errorcluster)  [unwired: 9 in]
                  }
                }
              }
              frame "/Temp", "/Temperature" {
                n217 = case shown="\"GET\"" w718 {
                  tunnel: [w723 w738] -> w722
                  tunnel: w721 -> [w727 w737]
                  tunnel: w720 -> [_ _]
                  tunnel: w719 -> [w726 w736]
                  tunnel: w717 -> [_ _]
                  tunnel: w716 -> [_ _]
                  frame Default {
                    w728 = u16 405  # Not Allowed
                    n218 = call "Set Status Code.vi"("error in (no error)"=w727, "Status Code"=w728, "Response in"=w726) -> ("error out"=w724:errorcluster, "Response out"=w725:refnum<class "Response.lvclass">)  [unwired: 7 in]
                    n219 = call "Send.vi"("error in (no error)"=w724, "Response in"=w725) -> ("error out"=w723:errorcluster)  [unwired: 9 in]
                  }
                  frame "GET" {
                    # "Send (success)\nResponse"
                    # "Get the Current Iron Block Temperature"
                    n220 = local read "Temperature"() -> (w735:dbl)
                    n221 = Format Into String(w735) -> (resulting string=w734:string)  [unwired: 3 in, 1 out]
                    n222 = call "Set Body.vi"("error in (no error)"=w737, "Body"=w734, "Response in"=w736) -> ("error out"=w732:errorcluster, "Response out"=w729:refnum<class "Response.lvclass">)  [unwired: 7 in]
                    n223 = call "Set Status Code.vi"("error in (no error)"=w732, "Status Code"=u16 200, "Response in"=w729) -> ("error out"=w731:errorcluster, "Response out"=w730:refnum<class "Response.lvclass">)  [unwired: 7 in]
                    n224 = call "Send.vi"("error in (no error)"=w731, "Response in"=w730) -> ("error out"=w738:errorcluster)  [unwired: 9 in]
                  }
                }
              }
              frame "/Target" {
                n225 = case shown="\"GET\"" w741 {
                  tunnel: [w746 w759 w771] -> w745
                  tunnel: w744 -> [w750 w757 w770]
                  tunnel: w743 -> [_ _ _]
                  tunnel: w742 -> [w749 w752 w769]
                  tunnel: w740 -> [_ w761 _]
                  tunnel: w739 -> [_ w758 _]
                  frame Default {
                    w751 = u16 405  # Not Allowed
                    n226 = call "Set Status Code.vi"("error in (no error)"=w750, "Status Code"=w751, "Response in"=w749) -> ("error out"=w747:errorcluster, "Response out"=w748:refnum<class "Response.lvclass">)  [unwired: 7 in]
                    n227 = call "Send.vi"("error in (no error)"=w747, "Response in"=w748) -> ("error out"=w746:errorcluster)  [unwired: 9 in]
                  }
                  frame "POST" {
                    # "Send (empty success)\nResponse"
                    # "Send Message to Process Loop to\nUpdate Target Temperature"
                    n228 = call-dynamic "Send Message.vi"("MLA"=w761, "Message"="Process.Target", "Param 1"=w758, "error in (no error)"=w757) -> ("error out"=w756:errorcluster)  [unwired: 14 in, 1 out]
                    n229 = call "Set Status Code.vi"("error in (no error)"=w756, "Status Code"=u16 200, "Response in"=w752) -> ("error out"=w753:errorcluster, "Response out"=w754:refnum<class "Response.lvclass">)  [unwired: 7 in]
                    n230 = call "Send.vi"("error in (no error)"=w753, "Response in"=w754) -> ("error out"=w759:errorcluster)  [unwired: 9 in]
                  }
                  frame "GET" {
                    # "Send (empty success)\nResponse"
                    # "Get the Current Ambient Temperature"
                    n231 = local read "Target"() -> (w768:dbl)
                    n232 = Format Into String(w768) -> (resulting string=w767:string)  [unwired: 3 in, 1 out]
                    n233 = call "Set Body.vi"("error in (no error)"=w770, "Body"=w767, "Response in"=w769) -> ("error out"=w762:errorcluster, "Response out"=w765:refnum<class "Response.lvclass">)  [unwired: 7 in]
                    n234 = call "Set Status Code.vi"("error in (no error)"=w762, "Status Code"=u16 200, "Response in"=w765) -> ("error out"=w763:errorcluster, "Response out"=w764:refnum<class "Response.lvclass">)  [unwired: 7 in]
                    n235 = call "Send.vi"("error in (no error)"=w763, "Response in"=w764) -> ("error out"=w771:errorcluster)  [unwired: 9 in]
                  }
                }
              }
              frame Default {
              }
            }
          }
          frame True {
            # "No REST Message"
          }
        }
      }
      frame "Initialize", "This.Initialize" {
      }
    }
    n236 = call "LogError.vi"("Error To Log"=w574, "Context (\"Error\")"="REST" ("Context"), "reference in"=w563) -> ("Cleaned Error"=w575:errorcluster, "Stop?"=w565:bool)  [unwired: 2 in, 1 out]
  }
  n237 = call "Listen.vi"("error in (no error)"=w21, "Listen Port (80)"=w7, "API Queue"=w20) -> ("error out"=w1:errorcluster)  [unwired: 8 in]
  n238 = call "Server_CleanUp.vi"("error in (no error)"=w1) -> ()  [unwired: 10 in, 1 out]
  n239 = for {
    tunnel: w17 -> [w776] mode=indexing
    tunnel: [w775] -> w15 mode=indexing
    n240 = call-dynamic "Destroy.vi"("reference in"=w776) -> ("error out"=w775:errorcluster)  [unwired: 9 in, 1 out]
  }
  n241 = Merge Errors(w16, w15) -> (w14:errorcluster)
  n242 = Merge Errors(w73, w2, w38, w14) -> (w28:errorcluster)
  n243 = call-dynamic "Destroy.vi"("MLA"=w40, "error in (no error)"=w28) -> ("error out"=w13:errorcluster)  [unwired: 16 in, 1 out]
  n244 = call <vilib>:"Clear Errors.vi"("error in (no error)"=w13) -> ("error out"=w39:errorcluster)  [unwired: 5 in, 1 out]
  n245 = property class="App"(error in=w39) -> ("App.Kind"=w72:T5)  [unwired: 1 in, 2 out]
  n246 = Equal?(x=w72, y=T5."Run Time System" ("Application:Kind")) -> (x = y?=w70:bool)
  n247 = Quit LabVIEW(quit? (T)=w70) -> ()
  "Version" <- w42
